vi "EvaluateAuthorizationExpression.vi"(8 "Error In":errorcluster, 10 "Expression":string, 11 "reference in":refnum<class "UserManager.lvclass">) -> (0 "Error Out":errorcluster, 1 "Result":T1, 2 "Pass":bool, 3 "reference in":refnum<class "UserManager.lvclass">)   [LabVIEW 2021, in "UserMananger.lvlib" / "UserManager.lvclass"]
uses:
  UserManager.lvclass
  Library_TAF_Support/Expressions/Expressions.lvlib
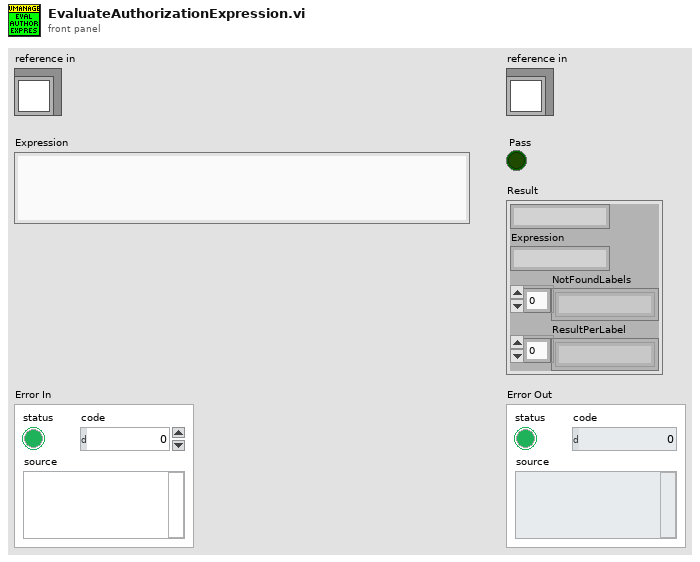
[diagram p1: front panel]
types:
  T1 = cluster{string, "Expression":string, "NotFoundLabels":string[], "ResultPerLabel":string[]}
  T2 = typedef "UserMananger.lvlib/UserManager.lvclass/ObjectAttributes.ctl" = cluster{"Interfaces":cluster{"ActivationUpdated":refnum<class "IAuthorizationUpdated.lvclass">}, "Locals":cluster{"MainGUIActive":refnum<queue>, "Evaluations":cluster{"Label":string, "Value":string}[]}, "Persistent":cluster{"Dummy":bool}}
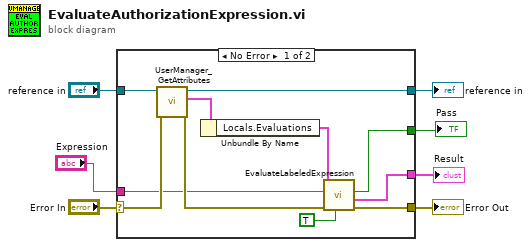
[diagram p0: block diagram]
diagram:
  n1 = case shown="No Error" "Error In" {
    selector: "Error In" -> [w18 w20]
    tunnel: [w12 w20] -> w6
    tunnel: [w15 w19] -> w4
    tunnel: "reference in" -> [w16 w19]
    tunnel: "Expression" -> [w10 _]
    tunnel: [w9 _] -> w2
    tunnel: [w8 _] -> w1
    frame No Error {
      n2 = call "UserManager_GetAttributes.vi"("error in (no error)"=w18, "reference in"=w16) -> ("error out"=w13:errorcluster, "Data"=w17:T2, "reference out"=w15:refnum<class "UserManager.lvclass">)  [unwired: 6 in, 1 out]
      n3 = Unbundle By Name(w17) -> ("Locals.Evaluations"=w11:cluster{"Label":string, "Value":string}[])
      n4 = call "EvaluateLabeledExpression.vi"("AllowMissingLabels"=TRUE, "error in (no error)"=w13, "Expression"=w10, "Labels"=w11) -> ("error out"=w12:errorcluster, "Log"=w8:T1, "Result"=w9:bool)  [unwired: 5 in]
    }
    frame Error {
    }
  }
  "Error Out" <- w6
  "reference in" <- w4
  "Pass" <- w2
  "Result" <- w1
